vi "Problem 3 - Largest prime factor.vi"() -> ()   [LabVIEW 2021, in "Project Euler.lvlib"]
uses:
  Project Euler.lvlib
  Utilities/Numeric Utilities/Numeric Utilities.lvlib
panel:
  out "All divisors of 600851475143":i32[](array[numeric])
  out "Number that can be represented in I32":i64
  out "divisors of 600851475143 that are less than 1000":i64[](array[numeric])
  out "Answer - largest divisor":i32
  # "Development\nControls or indicators that are useful for development or testing, but which are not outputs of the VI."
  # "Input\nInputs to the VI"
  # "Output\nOutputs of the VI"
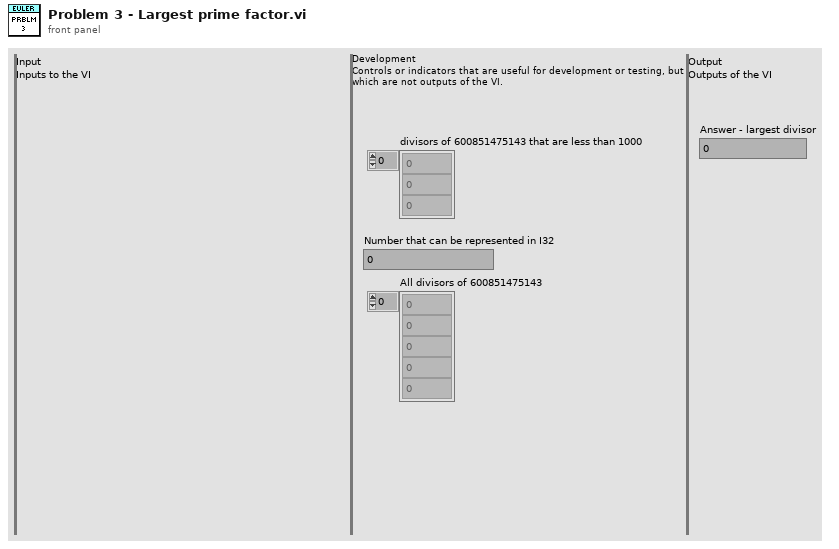
[diagram p1: front panel]
types:
  T1 = typedef "Numeric Utilities.lvlib/Factors cluster.ctl" = cluster{"Factor":i32, "Power":i32}
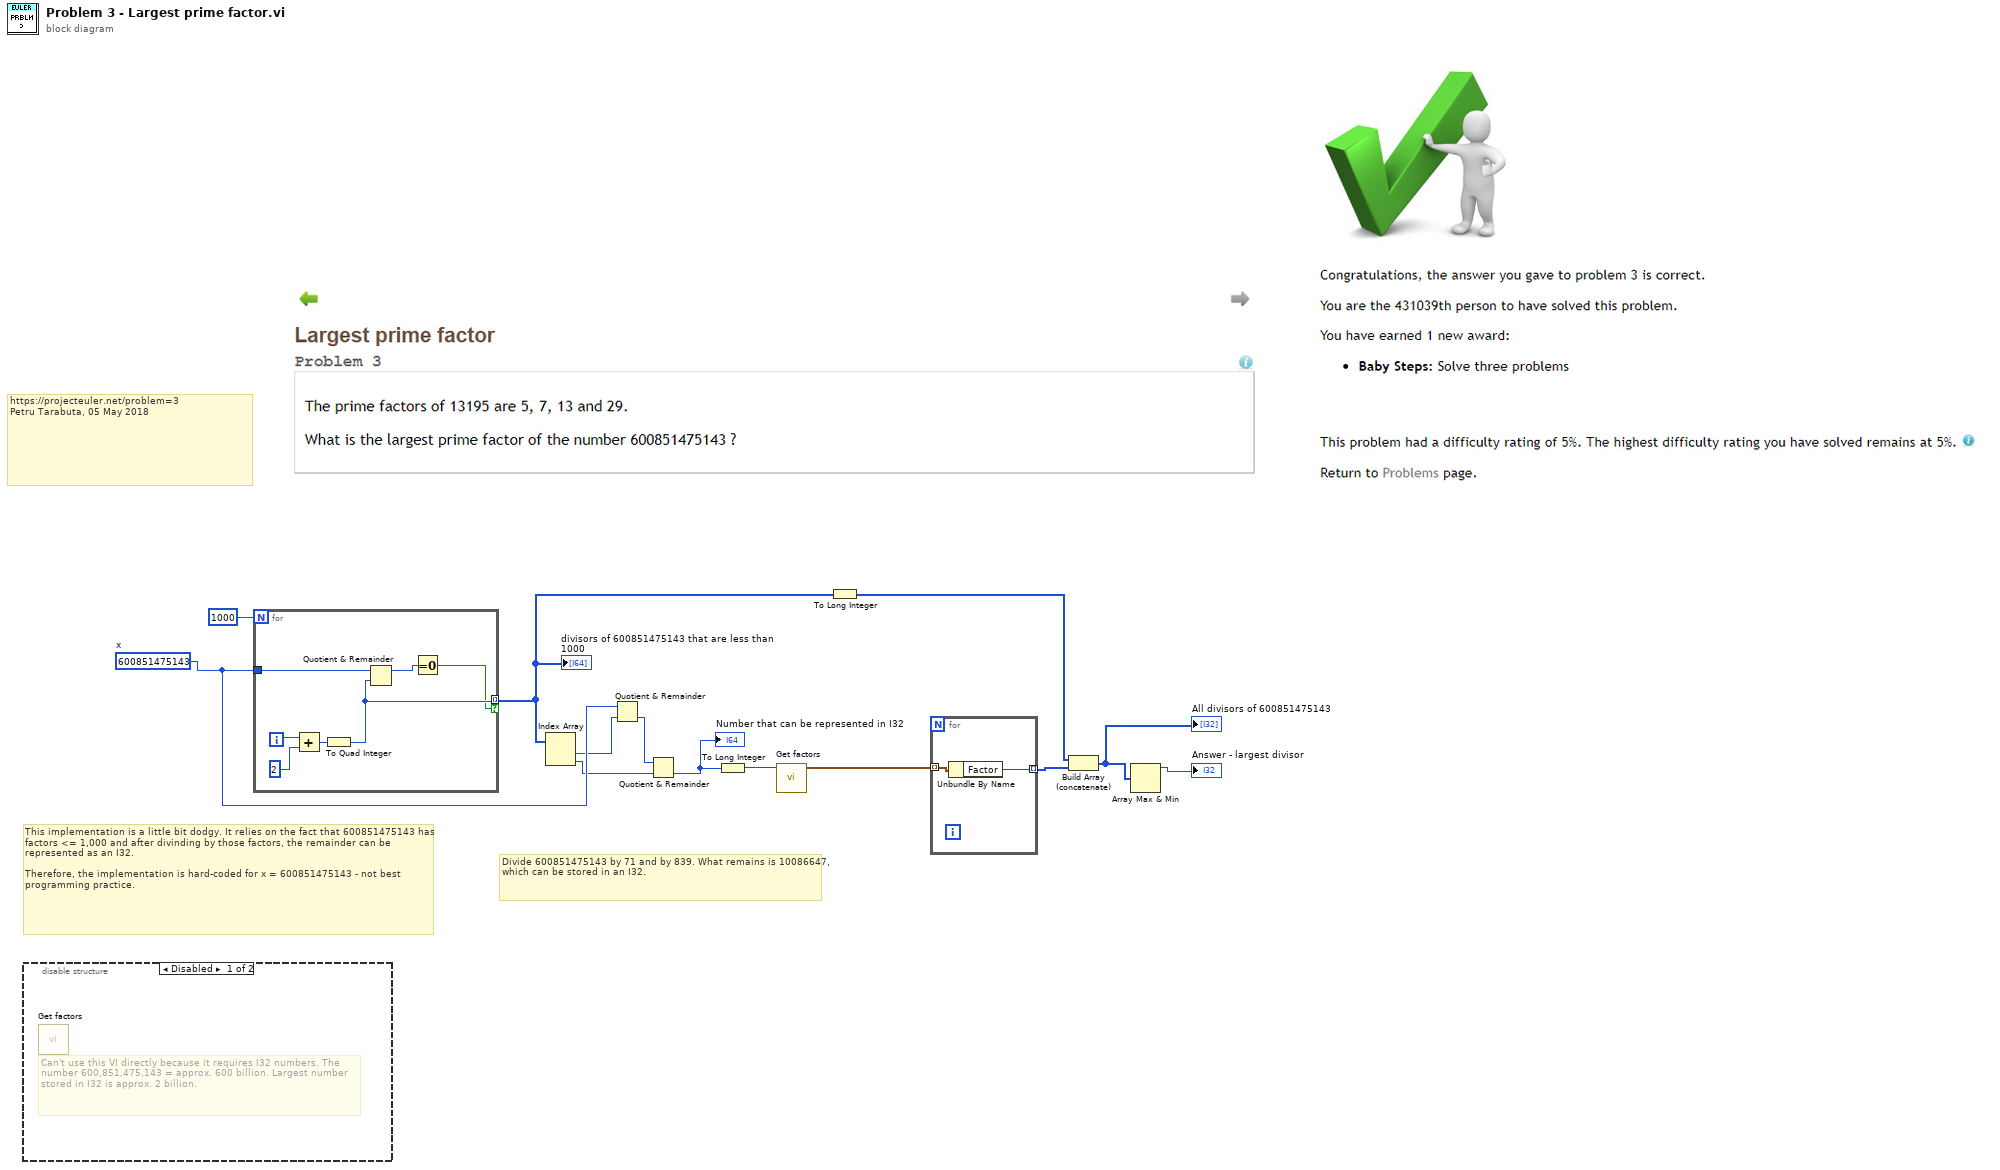
[diagram p0: block diagram]
diagram:
  w12 = i64 600851475143  # x
  # "This implementation is a little bit dodgy. It relies on the fact that 600851475143 has factors <= 1,000 and after divinding by those factors, the remainder can be represented as an I32.\n\nTherefore, the implementation is hard-coded for x = 600851475143 - not best programming practice."
  # "Divide 600851475143 by 71 and by 839. What remains is 10086647, which can be stored in an I32."
  # "https://projecteuler.net/problem=3\nPetru Tarabuta, 05 May 2018"
  n1 = disable-structure shown="Disabled" {
    frame Disabled {
      # "Can't use this VI directly because it requires I32 numbers. The number 600,851,475,143 = approx. 600 billion. Largest number stored in I32 is approx. 2 billion."
      n2 = call "Get factors.vi"() -> ()  [unwired: 6 in, 6 out]
    }
    frame Enabled {
    }
  }
  n3 = for {
    N: 1000 -> [_]
    tunnel: w12 -> [w20]
    tunnel: [w15] -> w4 mode=indexing if=w14
    i -> [w19]
    n4 = Add(x=w19, y=2) -> (x+y=w17:i32)
    n5 = To Quad Integer(1:w17) -> (0:w15:i64)
    n6 = Quotient & Remainder(x=w20, y=w15) -> (x-y*floor(x/y)=w16:i64)  [unwired: 1 out]
    n7 = Equal To 0?(x=w16) -> (x = 0?=w14:bool)
  }
  "divisors of 600851475143 that are less than 1000" <- w4
  n8 = Index Array(array=w4) -> (element #1=w11:i64, element #2=w10:i64)  [unwired: 2 in]
  n9 = Quotient & Remainder(x=w12, y=w11) -> (floor(x/y)=w9:i64)  [unwired: 1 out]
  n10 = Quotient & Remainder(x=w9, y=w10) -> (floor(x/y)=w8:i64)  [unwired: 1 out]
  "Number that can be represented in I32" <- w8
  n11 = To Long Integer(number=w8) -> (32bit integer=w7:i32)
  n12 = call "Get factors.vi"("x"=w7) -> ("Factors out"=w6:T1[])  [unwired: 5 in, 5 out]
  n13 = To Long Integer(number=w4) -> (32bit integer=w3:i32[])
  n14 = for {
    tunnel: w6 -> [w22] mode=indexing
    tunnel: [w21] -> w5 mode=indexing
    n15 = Unbundle By Name(w22) -> ("Factor"=w21:i32)
  }
  n16 = Build Array (concatenate)(w3, w5) -> (w2:i32[])
  "All divisors of 600851475143" <- w2
  n17 = Array Max & Min(array=w2) -> (max value=→"Answer - largest divisor":i32)  [unwired: 3 out]
